vi "GOMDBTS2048 get Color.vi"(0 "handle":i32, 11 "error in (no error)":errorcluster) -> (1 "domWL":dbl, 2 "vs":dbl, 3 "y":dbl, 4 "UpperX":dbl, 6 "UpperY":dbl, 8 "UpperZ":dbl, 10 "x":dbl, 12 "function return":i32, 13 "CCT":dbl, 14 "us":dbl, 15 "error out":errorcluster)   [LabVIEW 2015, in "GOMDBTS2048.lvlib"]
doc: "GOBTS2048DLL int __stdcall GOMDBTS2048_getColor(int handle, double* UpperX, double* UpperY, double* UpperZ, double* x, double* y,\n double* us, double* vs, double* CCT, double* domWL);"
uses:
  GOMDBTS2048.lvlib
  runtime/GOMDBTS2048.dll
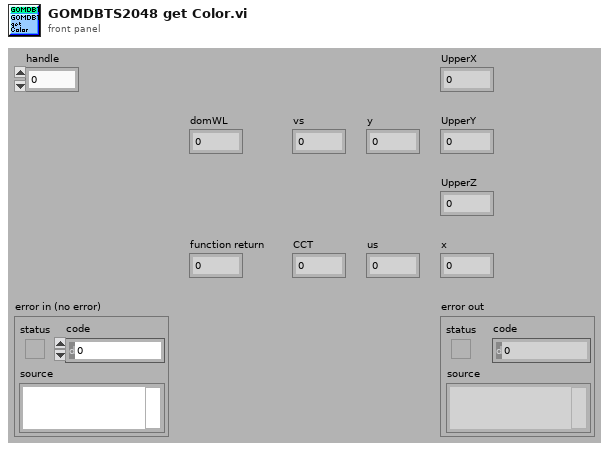
[diagram p1: front panel]
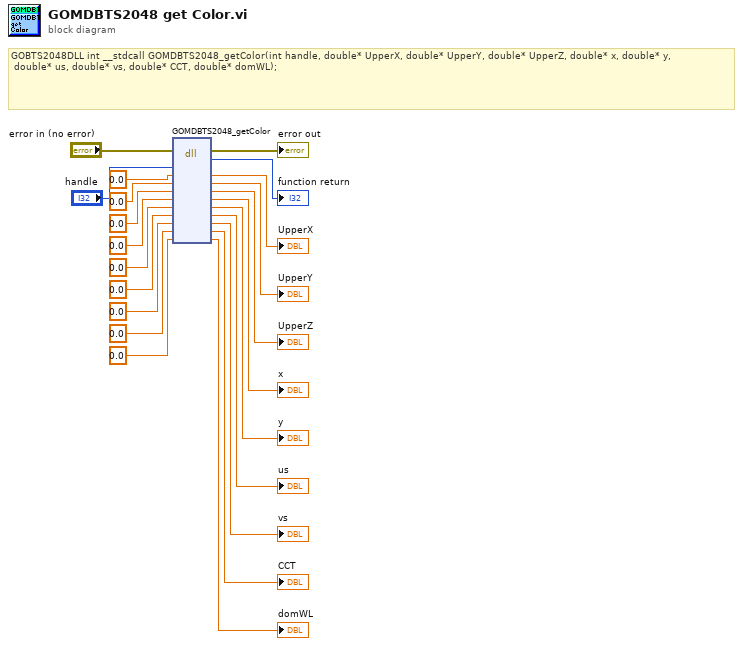
[diagram p0: block diagram]
diagram:
  # "GOBTS2048DLL int __stdcall GOMDBTS2048_getColor(int handle, double* UpperX, double* UpperY, double* UpperZ, double* x, double* y,\n\tdouble* us, double* vs, double* CCT, double* domWL);"
  n1 = dll-call lib="C:/Users/rkoch/Documents/GO_Library/runtime/GOMDBTS2048.*" fn="GOMDBTS2048_getColor"(error in="error in (no error)", "handle"="handle", "UpperX"=0.0, "UpperY"=0.0, "UpperZ"=0.0, "x"=0.0, "y"=0.0, "us"=0.0, "vs"=0.0, "CCT"=0.0, "domWL"=0.0) -> (error out=→"error out":errorcluster, →"function return":i32, "UpperX"=→"UpperX":dbl, "UpperY"=→"UpperY":dbl, "UpperZ"=→"UpperZ":dbl, "x"=→"x":dbl, "y"=→"y":dbl, "us"=→"us":dbl, "vs"=→"vs":dbl, "CCT"=→"CCT":dbl, "domWL"=→"domWL":dbl)  [unwired: 3 in, 1 out]
